vi "SetExtAcquisition.vi"(8 "error in (no error)":errorcluster, 10 "ExtAcquisition":T1, 11 "ScopePluginsBase in":refnum<class "ScopePluginsBase.lvclass">) -> (0 "error out":errorcluster, 3 "ScopePluginsBase out":refnum<class "ScopePluginsBase.lvclass">)   [LabVIEW 2014, in "ScopePlugins.lvlib" / "ScopePluginsBase.lvclass"]
uses:
  ScopePluginsBase.lvclass
  InfiniiumClass/Typedefs/ExtAcquisition.ctl
  InfiniiumClass/Infiniium.lvclass
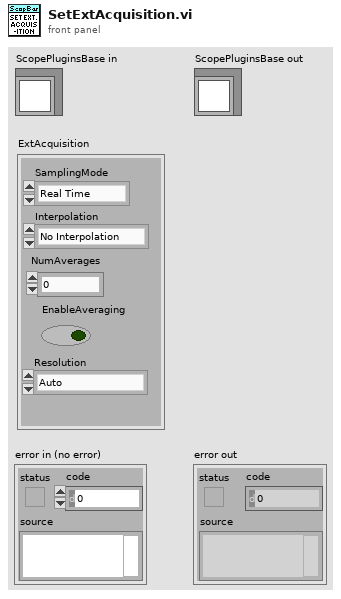
[diagram p1: front panel]
types:
  T1 = typedef "ScopePlugins.lvlib/Infiniium.lvclass/ExtAcquisition.ctl" = cluster{"SamplingMode ":enum16{"Real Time", "Equivalent Time", "Segment", "Real Time Peak Detect", "Real Time High Resolution", "Peak Detect Segment", "High Resolution Segment"}, "Interpolation":enum16{"No Interpolation", "sin(x)/x", "1 Point sin(x)/x", "2 Point sin(x)/x", "4 Point sin(x)/x", "8 Point sin(x)/x", "16 Point sin(x)/x"}, "NumAverages":i32, "EnableAveraging":bool, "Resolution":enum16{"Auto", "Bits 9", "Bits 10", "Bits 11", "Bits 12"}}
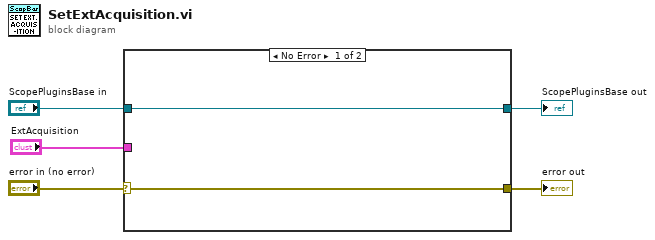
[diagram p0: block diagram]
diagram:
  n1 = case shown="No Error" "error in (no error)" {
    selector: "error in (no error)" -> [w6 w9]
    tunnel: [w6 w9] -> w4
    tunnel: [w7 w8] -> w2
    tunnel: "ScopePluginsBase in" -> [w7 w8]
    tunnel: "ExtAcquisition" -> [_ _]
    frame No Error {
    }
    frame Error {
    }
  }
  "error out" <- w4
  "ScopePluginsBase out" <- w2
